vi "Add SLSC Switch Custom Device.vi"(8 "error in":errorcluster, 10 "slot number":u32=1, 11 "slsc chassis in":T1 format="%.0x") -> (0 "error out":errorcluster, 2 "slsc switch custom device":T1 format="%.0x", 3 "slsc chassis out":T1 format="%.0x")   [LabVIEW 2017, in "NI-SWITCH Scripting.lvlib"]
doc: "Creates and adds a new instance of the SLSC Switch custom device to the SLSC chassis in the specified slot."
uses:
  NI-SWITCH Scripting.lvlib
  Shared/VeriStand SLSC Scripting/VeriStand SLSC Scripting.lvlib
  SLSC Scripting Constants.vi
  NationalInstruments.VeriStand.SystemStorage
  <vilib>/NI Veristand/Custom Device API/Custom Device Item Ref.ctl
  <vilib>/NI VeriStand/Custom Device API/Custom Device API.lvlib
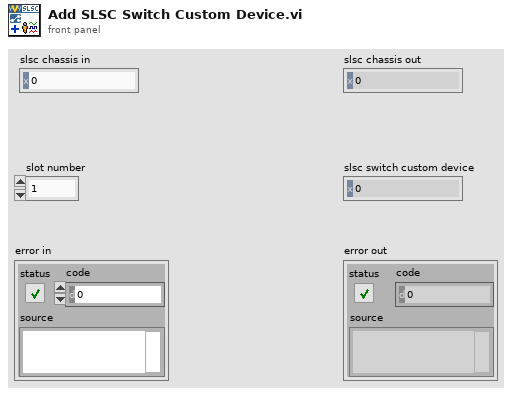
[diagram p1: front panel]
types:
  T1 = typedef "Custom Device API.lvlib/Custom Device Item Ref.ctl" = u64
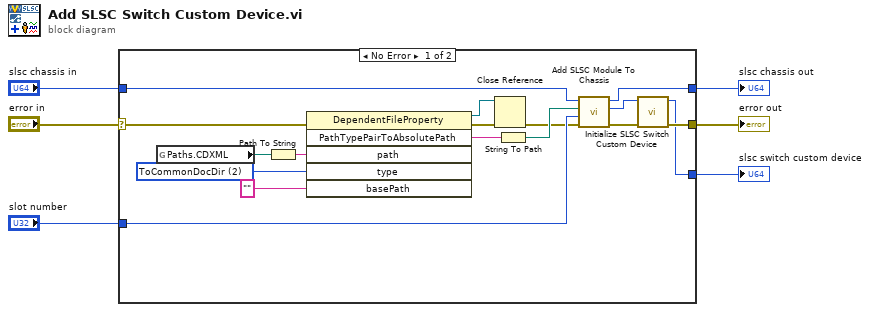
[diagram p0: block diagram]
diagram:
  n1 = case shown="No Error" "error in" {
    selector: "error in" -> [w14 w24]
    tunnel: "slsc chassis in" -> [w17 _]
    tunnel: [w16 _] -> w2
    tunnel: "slot number" -> [w15 _]
    tunnel: [w10 w24] -> w5
    tunnel: [w7 _] -> w3
    frame No Error {
      w23 = 2 items=["Absolute", "Relative", "ToCommonDocDir", "ToApplicationDataDir"] ("type")
      n2 = global read "SLSC Scripting Constants.vi" "Paths.CDXML"() -> (w19:path)
      n3 = Path To String(path=w19) -> (string=w21:string)
      n4 = invoke class="DependentFileProperty" method="PathTypePairToAbsolutePath"(error in=w14, "path"=w21, "type"=w23, "basePath"="") -> (reference out=w11:refnum<k24>, error out=w13:errorcluster, "PathTypePairToAbsolutePath"=w20:string)  [unwired: 2 in, 3 out]
      n5 = Close Reference(reference=w11, error in (no error)=w13) -> (error out=w12:errorcluster)
      n6 = String To Path(string=w20) -> (path=w18:path)
      n7 = call "Add SLSC Module To Chassis.vi"("error in (no error)"=w12, "Slot Number"=w15, "SLSC Custom Device XML"=w18, "SLSC Chassis"=w17) -> ("error out"=w9:errorcluster, "SLSC Module"=w8:u64, "SLSC Chassis out"=w16:u64)  [unwired: 5 in]
      n8 = call "Initialize SLSC Switch Custom Device.vi"("error in"=w9, "slsc switch custom device in"=w8) -> ("error out"=w10:errorcluster, "slsc switch custom device out"=w7:T1)  [unwired: 7 in, 1 out]
    }
    frame Error {
    }
  }
  "error out" <- w5
  "slsc switch custom device" <- w3
  "slsc chassis out" <- w2
